vi "GenNet Init Client.vi"(4 "Module Timeout":i32, 6 "System Message":refnum<user-event>, 7 "GenNet-Client ID":i32, 8 "error in (no error)":errorcluster, 9 "Port Number":u16, 10 "IP Address":string, 11 "DQMH-GenNet Message Queue in":refnum<class "DQMH-GenNet Message Queue.lvclass">) -> (0 "error out":errorcluster, 3 "DQMH-GenNet Message Queue out":refnum<class "DQMH-GenNet Message Queue.lvclass">, 5 "GenNet-Client ID out":i32)   [LabVIEW 2020, in "hse-gennet.lvlib"]
doc: "Initializes a GenNet Client if <B>ClientID == -1</B> and automatically connects to it. See usage example inside for how to use this VI.\n\n____\nHAMPEL SOFTWARE ENGINEERING v3.8.0 (2023-12-18 14:41)"
uses:
  hse-gennet.lvlib
  hse-dqmh/Controls/System Message Argument--cluster.ctl
  hse-dqmh/Controls/System Message Source.ctl
  DQMH-GenNet Message Queue.lvclass
  DQMH-GenNet Message Queue.lvclass/DQMH-GenNet Message Queue.ctl
  GenNet-Client/GenNet-Client.lvlib
  GenNet-Client/Clone Registration/Clone Registration.lvlib
  hse-dqmh/hse-dqmh.lvlib
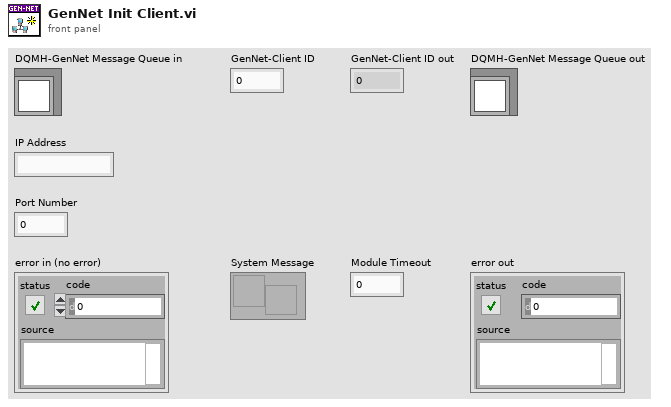
[diagram p1: front panel]
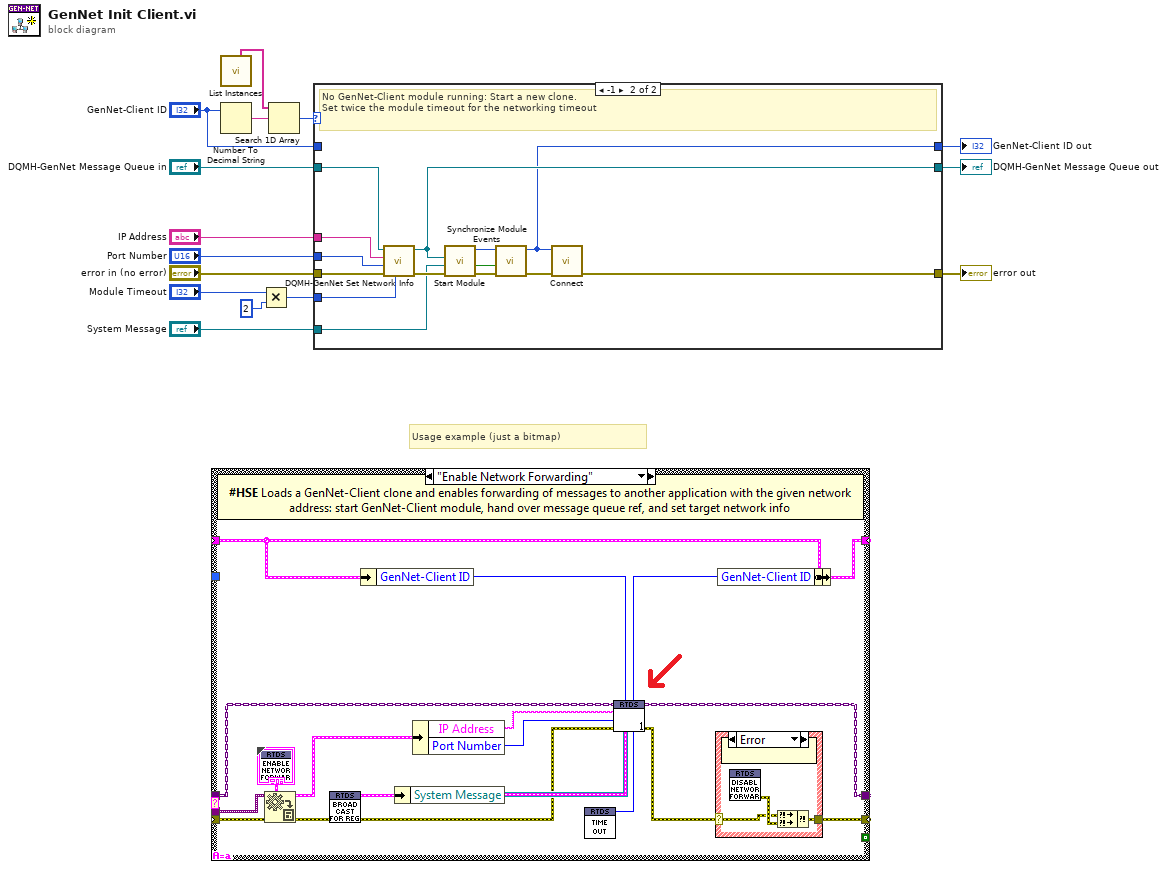
[diagram p0: block diagram]
diagram:
  # "Usage example (just a bitmap)"
  n1 = call "List Instances.vi"() -> ("Instances Names"=w9:string[])  [unwired: 7 in, 4 out]
  n2 = Number To Decimal String(number="GenNet-Client ID") -> (decimal integer string=w7:string)  [unwired: 1 in]
  n3 = Multiply(x="Module Timeout", y=2) -> (x*y=w2:i32)
  n4 = Search 1D Array(1D array=w9, element=w7) -> (index of element=w8:i32)  [unwired: 1 in]
  n5 = case shown="-1" w8 {
    tunnel: [w18 w26] -> w4
    tunnel: [w17 w21] -> w5
    tunnel: "error in (no error)" -> [w17 w28]
    tunnel: "DQMH-GenNet Message Queue in" -> [w18 w29]
    tunnel: "System Message" -> [_ w25]
    tunnel: [w16 w20] -> w12
    tunnel: "GenNet-Client ID" -> [w16 _]
    tunnel: "Port Number" -> [_ w24]
    tunnel: "IP Address" -> [_ w23]
    tunnel: w2 -> [_ w19]
    frame Default {
      # "GenNet-Client clone already running..."
    }
    frame -1 {
      # "No GenNet-Client module running: Start a new clone.\nSet twice the module timeout for the networking timeout"
      n6 = call "DQMH-GenNet Set Network Info.vi"("Timeout (default 5000ms)"=w19, "error in (no error)"=w28, "Port Number"=w24, "IP Address"=w23, "Message Queue in"=w29) -> ("error out"=w27:errorcluster, "Message Queue out"=w26:refnum<class "DQMH-GenNet Message Queue.lvclass">)  [unwired: 5 in]
      n7 = call "Start Module.vi"("error in (no error)"=w27, "Caller SystemMsg"=w25, "Caller MsgQ"=w26) -> ("error out"=w32:errorcluster, "Wait for Event Sync?"=w31:bool, "Module ID"=w30:i32)  [unwired: 5 in, 1 out]
      n8 = call "Synchronize Module Events.vi"("error in (no error)"=w32, "Wait for Event Sync?"=w31, "Module ID"=w30) -> ("error out"=w22:errorcluster, "Module ID (dup)"=w20:i32)  [unwired: 7 in]
      n9 = call "Connect.vi"("error in (no error)"=w22, "Module ID"=w20) -> ("error out"=w21:errorcluster)  [unwired: 8 in, 1 out]
    }
  }
  "GenNet-Client ID out" <- w12
  "error out" <- w5
  "DQMH-GenNet Message Queue out" <- w4
